vi "Create Event Reg.vi"(8 "error in (no error)":errorcluster, 9 "Method Names":string[](array[string]), 10 "Object Name":string, 11 "JKI_Python_Server in":refnum<class "Server.lvclass">) -> (0 "error out":errorcluster, 1 "Python":T1, 3 "JKI_Python_Server out":refnum<class "Server.lvclass">)   [LabVIEW 2013, in "JKI_Python_Bridge_for_LV.lvlib" / "Server.lvclass"]
uses:
  Server.lvclass
  Type Definitions/Python Method Call - Event Registration.ctl
  Call/Call.lvclass
  Type Definitions/Public Events - Cluster.ctl
  CallHandler/CallHandler.lvclass
  CallHandler/CallHandler.lvclass/CallHandler.ctl
  Server.lvclass/Server.ctl
  Type Definitions/Python Node.ctl
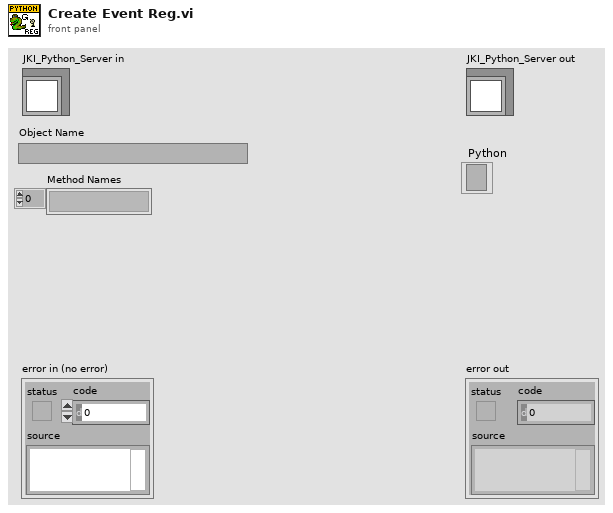
[diagram p1: front panel]
types:
  T1 = typedef "JKI_Python_Bridge_for_LV.lvlib/Server.lvclass/Python Method Call - Event Registration.ctl" = refnum<event-registration>
  T2 = typedef "JKI_Python_Bridge_for_LV.lvlib/Server.lvclass/Python Node.ctl" = cluster{"Name":string, "Python Method Call":refnum<user-event>, "Call Handle":refnum<class "CallHandler.lvclass">}
  T3 = typedef "JKI_Python_Bridge_for_LV.lvlib/Server.lvclass/Public Events - Cluster.ctl" = cluster{"Stop Nodes":refnum<user-event>}
  T4 = typedef "JKI_Python_Bridge_for_LV.lvlib/Server.lvclass/Class Private Data - Cluster.ctl" = cluster{"TCP Server RefNum":T5, "TCP port (50007)":u16, "max connections (0: no limit)":u32, "net address (0: Listen on All Adaptors)":u32, "Nodes":T2[], "Public Events":T3}
  T5 = typedef "TCP Server Object RefNum__jki_lib_tcp_server.ctl" = refnum<k1>
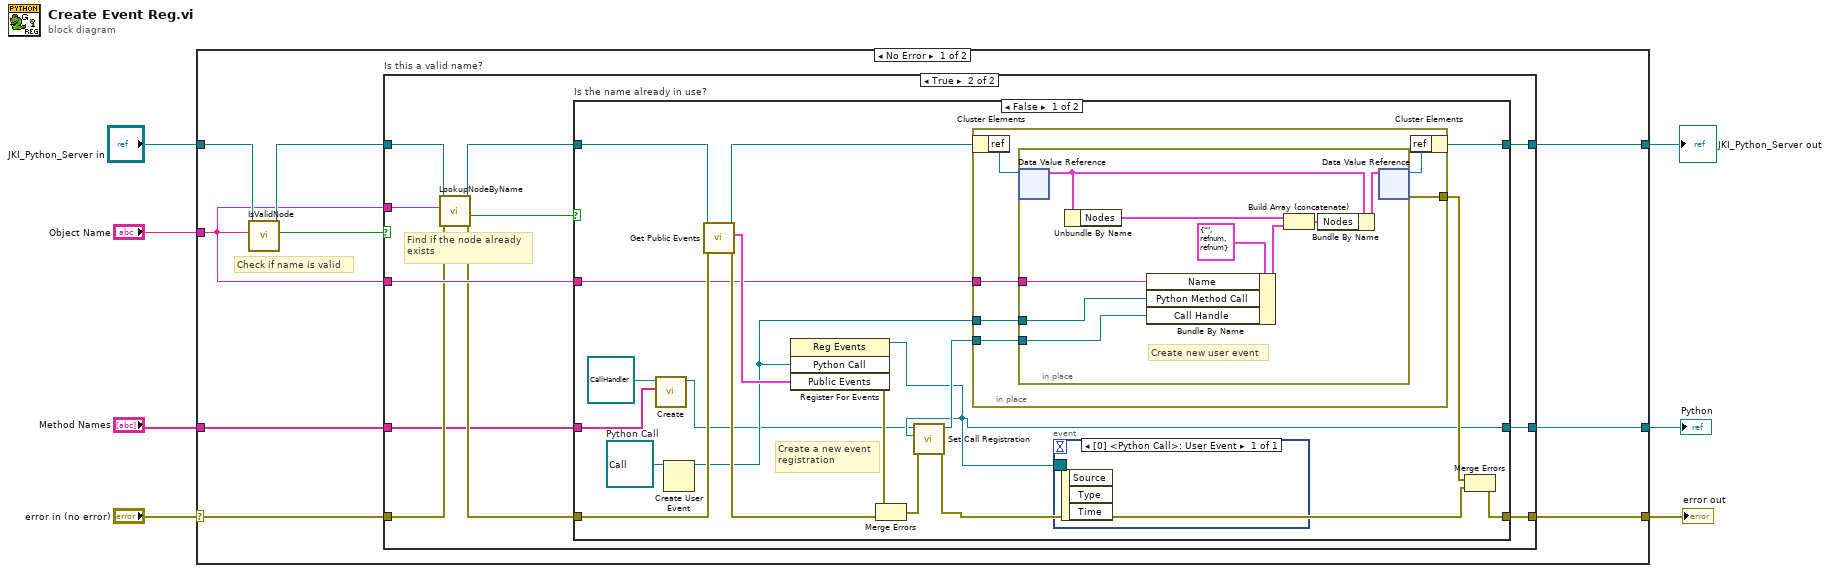
[diagram p0: block diagram]
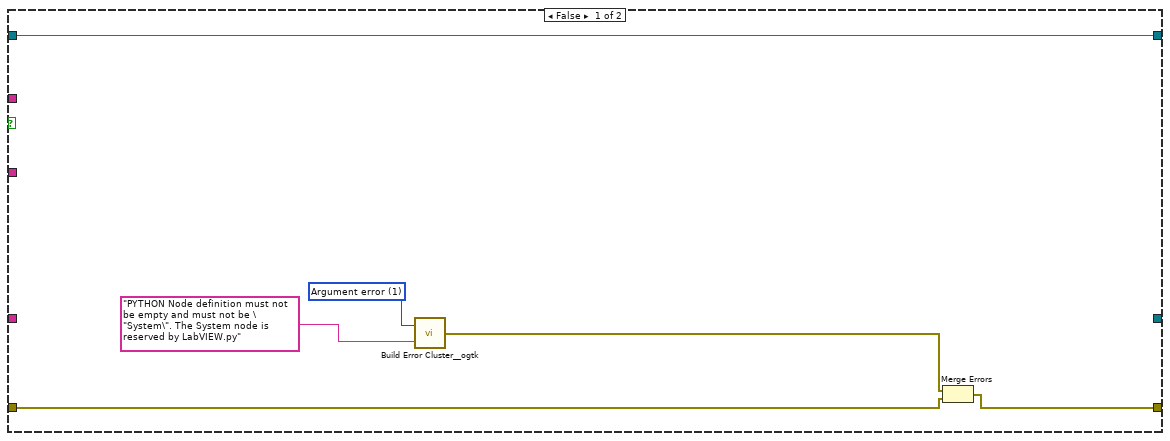
[diagram p2: hidden frame]
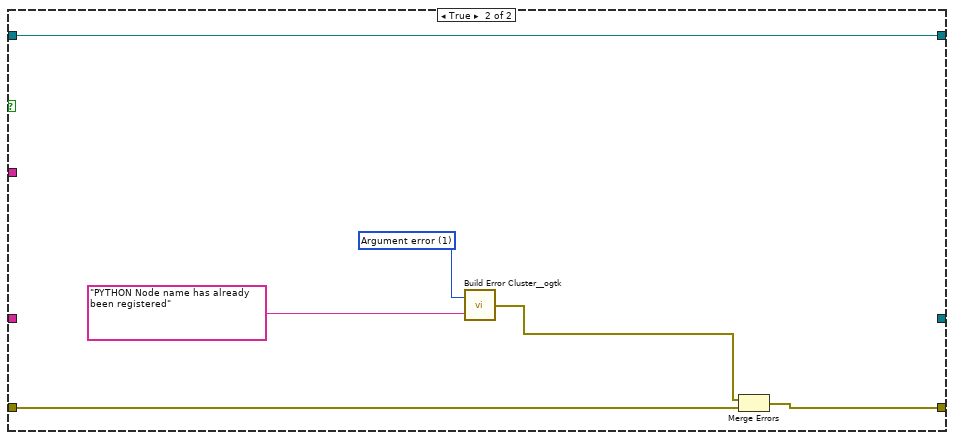
[diagram p3: hidden frame]
diagram:
  n1 = case shown="No Error" "error in (no error)" {
    selector: "error in (no error)" -> [w11 w75]
    tunnel: [w10 w75] -> w6
    tunnel: [w12 w74] -> w4
    tunnel: "JKI_Python_Server in" -> [w16 w74]
    tunnel: [w8 _] -> w3
    tunnel: "Method Names" -> [w9 _]
    tunnel: "Object Name" -> [w13 _]
    frame No Error {
      # "Check if name is valid"
      n2 = call "IsValidNode.vi"("Node Name"=w13, "Server in"=w16) -> ("Valid Node Definition?"=w14:bool, "Server out"=w15:refnum<class "Server.lvclass">)  [unwired: 8 in]
      n3 = case "Is this a valid name?" shown="True" w14 {
        tunnel: w15 -> [w20 w31]
        tunnel: w13 -> [_ w33]
        tunnel: [w20 w32] -> w12
        tunnel: w13 -> [_ w28]
        tunnel: [_ w27] -> w8
        tunnel: w11 -> [w18 w26]
        tunnel: [w17 w24] -> w10
        tunnel: w9 -> [_ w23]
        frame False {
          w21 = 1 items=["No error", "Argument error", "Memory is full", "Out of zone", "End of file", "File already open", "Generic file I/O error", "File not found", "File permission error", "Disk is full", "Duplicate path", "Too many files open", "System feature not enabled", "Resource file not found", "Cannot add resource", "Resource not found", "Image not found", "Image memory error", "Pen does not exist", "Config type invalid", "Config token not found", "Config parse error", "Config memory error", "Bad external code format", "Bad external code offset", "External code not present", "Null window", "Destroy window error", "Null menu", "Print aborted", "Bad print record", "Print driver error", "Windows error during printing", "Memory error during printing", "Print dialog error", "Generic print error", "Invalid device refnum", "Device not found", "Device parameter error", "Device unit error", "Cannot open device", "Device call aborted", "Generic error", "Cancelled by user", "Object ID too low", "Object ID too high", "Object not in heap", "Unknown heap", "Unknown object (invalid DefProc)", "Unknown object (DefProc not in table)", "Message out of range", "Invalid (null) method", "Unknown message", "Manager call not supported", "Bad address", "Network operation in progress", "Network operation timed out", "Connection is busy", "Network attribute not supported", "Network error", "Address in use", "System out of memory", "Connection aborted", "Connection refused", "Not connected", "Already connected", "Connection closed", "Initialization error (interapplication manager)", "Bad occurrence", "Wait on unbound occurrence handler", "Occurrence queue overflow", "Datalog type conflict", "Unused", "Unrecognized type (interapplication manager)", "Memory corrupt", "Failed to make temporary DLL", "Old CIN version", "Drag socket not found", "Failed to load drop-object", "Failed to register OLE object", "Failed to release OLE object", "Format specifier type mismatch", "Unknown format specifier", "Too few format specifiers", "Too many format specifiers", "Scan failed", "Newer CIN version", "Error converting to variant", "Runtime menu error", "Password tampered", "Variant attribute not found", "Incompatible variant data type", "Event data is not available", "Event Store is not present", "Occurrence is not found", "Event Queue is not created", "Event info is not available", "Refnum passed is NULL", "Error retrieving Class GUID", "Error retrieving CoClass GUID", "Error retrieving TypeLib GUID.", "Bad built application magic bytes.", "Specific driver is different from the specific driver associated with the Logical Name.", "There is no session opened to the class driver.", "Max Error", "MAX - Error with config objects", "MAX - Error loading configuration", "MAX - Group not supported"]
          n4 = call <userlib>:"Build Error Cluster__ogtk.vi"("String to Prepend to source (\"\")"="PYTHON Node definition must not be empty and must not be \"System\". The System node is reserved by LabVIEW.py", "code"=w21) -> ("error out"=w19:errorcluster)
          n5 = Merge Errors(w19, w18) -> (w17:errorcluster)
        }
        frame True {
          # "Find if the node already\nexists"
          n6 = call "LookupNodeByName.vi"("error in (no error)"=w26, "Python Node Name"=w33, "Server in"=w31) -> ("error out"=w25:errorcluster, "Found?"=w29:bool, "Server out"=w30:refnum<class "Server.lvclass">)  [unwired: 5 in, 1 out]
          n7 = case "Is the name already in use?" shown="False" w29 {
            tunnel: [w44 w71] -> w32
            tunnel: w30 -> [w46 w71]
            tunnel: w28 -> [w43 _]
            tunnel: [w37 _] -> w27
            tunnel: w25 -> [w49 w69]
            tunnel: [w38 w68] -> w24
            tunnel: w23 -> [w35 _]
            frame False {
              w47 = refnum<class "Call.lvclass"> refnum  # Python Call
              # "Create a new event\nregistration"
              n8 = call "Create.vi"("Method List (Enum or Str Array)"=w35, "Node in"=refnum<class "CallHandler.lvclass"> refnum ("JKI_Python_Bridge_for_LV.lvlib:Node.lvclass")) -> ("Node out"=w34:refnum<class "CallHandler.lvclass">)  [unwired: 8 in, 1 out]
              n9 = Create User Event(user event datatype=w47) -> (user event=w42:refnum<user-event>)  [unwired: 1 in, 1 out]
              n10 = call "Get Public Events.vi"("error in (no error)"=w49, "JKI_Python_Server in"=w46) -> ("error out"=w48:errorcluster, "Public Events"=w50:T3, "JKI_Python_Server out"=w45:refnum<class "Server.lvclass">)  [unwired: 7 in]
              n11 = register-events(w42, w50) -> (reference out=w37:refnum<event-registration>, error out=w52:errorcluster)  [unwired: 2 in]
              n12 = Merge Errors(w52, w48) -> (w51:errorcluster)
              n13 = call "Set Call Registration.vi"("error in (no error)"=w51, "Call Registration"=w37, "Node in"=w34) -> ("error out"=w39:errorcluster, "Node out"=w41:refnum<class "CallHandler.lvclass">)  [unwired: 7 in]
              n14 = in-place {
                in-place-border: w43 -> [w56]
                in-place-border: [w55] -> w40
                in-place-border: w42 -> [w54]
                in-place-border: w41 -> [w53]
                n15 = in-place-cluster #1(w45) -> ("ref"=w58:refnum<data-value>)
                n16 = in-place {
                  in-place-border: w56 -> [w62]
                  in-place-border: w54 -> [w61]
                  in-place-border: w53 -> [w60]
                  # "Create new user event"
                  n17 = in-place-dvr #2(w58) -> (w66:T4)  [unwired: 1 out]
                  n18 = Unbundle By Name(w66) -> ("Nodes"=w65:T2[])
                  n19 = Bundle By Name(cluster=T2 {"Name"="", "Python Method Call"=refnum, "Call Handle"=refnum} ("PYTHON Node"), "Name"=w62, "Python Method Call"=w61, "Call Handle"=w60) -> (w59:T2)
                  n20 = Build Array (concatenate)(w65, w59) -> (w64:T2[])
                  n21 = Bundle By Name(cluster=w66, "Nodes"=w64) -> (w67:T4)
                  n22 = in-place-dvr #2(w67) -> (w57:refnum<data-value>, w55:errorcluster)
                }
                n23 = in-place-cluster #1("ref"=w57) -> (w44:refnum<class "Server.lvclass">)
              }
              n24 = event shown="[0] <Python Call>: User Event" {
                selector: w37 -> [_]
                dyn-events: _ -> [_]
                timeout: _ -> [_]
                event User Event {
                  n25 = event-data() -> ()  [unwired: 1 in, 3 out]
                }
              }
              n26 = Merge Errors(w40, w39) -> (w38:errorcluster)
            }
            frame True {
              w72 = 1 items=["No error", "Argument error", "Memory is full", "Out of zone", "End of file", "File already open", "Generic file I/O error", "File not found", "File permission error", "Disk is full", "Duplicate path", "Too many files open", "System feature not enabled", "Resource file not found", "Cannot add resource", "Resource not found", "Image not found", "Image memory error", "Pen does not exist", "Config type invalid", "Config token not found", "Config parse error", "Config memory error", "Bad external code format", "Bad external code offset", "External code not present", "Null window", "Destroy window error", "Null menu", "Print aborted", "Bad print record", "Print driver error", "Windows error during printing", "Memory error during printing", "Print dialog error", "Generic print error", "Invalid device refnum", "Device not found", "Device parameter error", "Device unit error", "Cannot open device", "Device call aborted", "Generic error", "Cancelled by user", "Object ID too low", "Object ID too high", "Object not in heap", "Unknown heap", "Unknown object (invalid DefProc)", "Unknown object (DefProc not in table)", "Message out of range", "Invalid (null) method", "Unknown message", "Manager call not supported", "Bad address", "Network operation in progress", "Network operation timed out", "Connection is busy", "Network attribute not supported", "Network error", "Address in use", "System out of memory", "Connection aborted", "Connection refused", "Not connected", "Already connected", "Connection closed", "Initialization error (interapplication manager)", "Bad occurrence", "Wait on unbound occurrence handler", "Occurrence queue overflow", "Datalog type conflict", "Unused", "Unrecognized type (interapplication manager)", "Memory corrupt", "Failed to make temporary DLL", "Old CIN version", "Drag socket not found", "Failed to load drop-object", "Failed to register OLE object", "Failed to release OLE object", "Format specifier type mismatch", "Unknown format specifier", "Too few format specifiers", "Too many format specifiers", "Scan failed", "Newer CIN version", "Error converting to variant", "Runtime menu error", "Password tampered", "Variant attribute not found", "Incompatible variant data type", "Event data is not available", "Event Store is not present", "Occurrence is not found", "Event Queue is not created", "Event info is not available", "Refnum passed is NULL", "Error retrieving Class GUID", "Error retrieving CoClass GUID", "Error retrieving TypeLib GUID.", "Bad built application magic bytes.", "Specific driver is different from the specific driver associated with the Logical Name.", "There is no session opened to the class driver.", "Max Error", "MAX - Error with config objects", "MAX - Error loading configuration", "MAX - Group not supported"]
              n27 = call <userlib>:"Build Error Cluster__ogtk.vi"("String to Prepend to source (\"\")"="PYTHON Node name has already been registered", "code"=w72) -> ("error out"=w70:errorcluster)
              n28 = Merge Errors(w70, w69) -> (w68:errorcluster)
            }
          }
        }
      }
    }
    frame Error {
    }
  }
  "error out" <- w6
  "JKI_Python_Server out" <- w4
  "Python" <- w3
